vi "subvi_sample_setting.vi"(7 "采样频率":dbl=50000.0 format="%0.2f", 8 "error in":errorcluster caption="错误输入", 11 "physical channel":string="PXI_4499_1/ai0") -> (0 "error out":errorcluster caption="错误输出", 3 "task out":refnum<k21> caption="任务输出")   [LabVIEW 2014]
uses:
  <vilib>/DAQmx/configure/timing.llb/DAQmx Timing (Sample Clock).vi
  <vilib>/DAQmx/create/channels.llb/DAQmx Create Channel (AI-Sound Pressure-Microphone).vi
  <resource>/objmgr/daqmx.rc
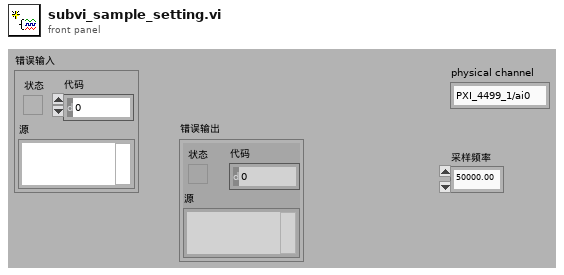
[diagram p1: front panel]
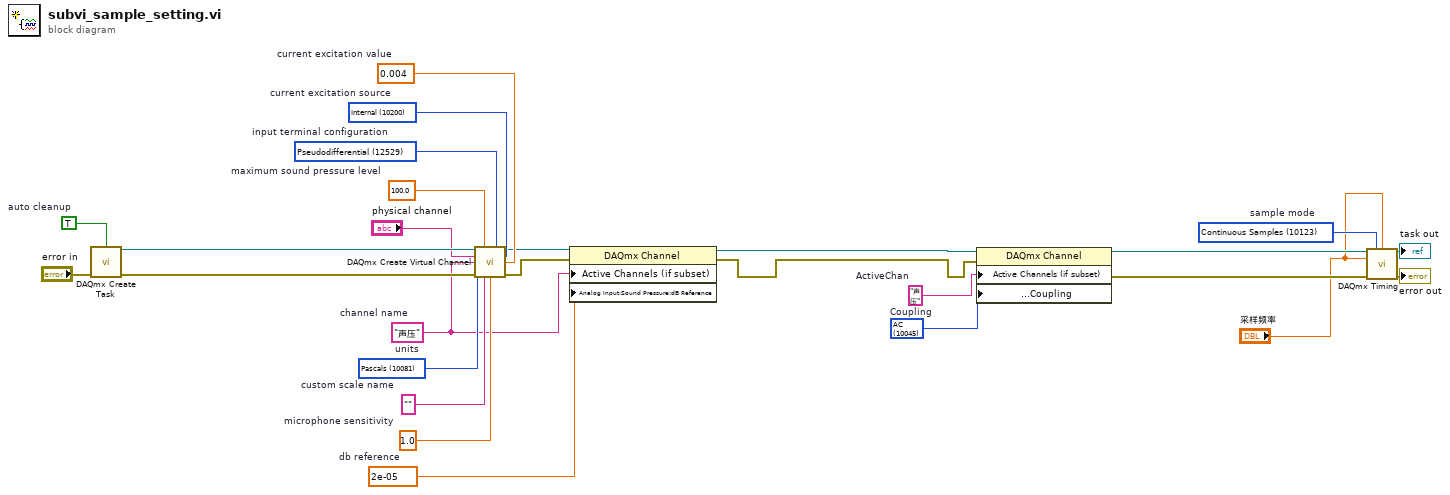
[diagram p0: block diagram]
diagram:
  w2 = 10123 items=["Finite Samples"=10178, "Continuous Samples"=10123, "Hardware Timed Single Point"=12522]  # sample mode
  w8 = 10045 items=["AC"=10045, "DC"=10050, "GND"=10066]  # Coupling
  w9 = "声压"  # ActiveChan
  w11 = 2e-05  # db reference
  w15 = 12529 items=["default"=-1, "RSE"=10083, "NRSE"=10078, "Differential"=10106, "Pseudodifferential"=12529]  # input terminal configuration
  w16 = 10081 items=["Pascals"=10081, "From Custom Scale"=10065]  # units
  w17 = 1.0  # microphone sensitivity
  w18 = 0.004  # current excitation value
  w19 = 10200 items=["Internal"=10200, "External"=10167, "None"=10230]  # current excitation source
  w20 = 100.0  # maximum sound pressure level
  w10 = "声压"  # channel name
  w21 = ""  # custom scale name
  w24 = TRUE  # auto cleanup
  n1 = call <vilib>:"DAQmx Create Task.vi"("auto cleanup"=w24, "error in"="error in") -> ("task out"=w23:refnum<k21>, "error out"=w25:errorcluster)  [unwired: 12 in]
  n2 = call-poly <vilib>:"DAQmx Create Virtual Channel.vi"("task in"=w23, "maximum sound pressure level"=w20, "input terminal configuration"=w15, "physical channels"="physical channel", "current excitation source"=w19, "name to assign"=w10, "current excitation value"=w18, "units"=w16, "error in"=w25, "custom scale name"=w21, "microphone sensitivity"=w17) -> ("task out"=w14:refnum<k21>, "error out"=w13:errorcluster)  [unwired: 3 in]
  n3 = property class="DAQmx Channel"(reference=w14, error in=w13, "Active Channels (if subset)"=w10, "Analog Input:Sound Pressure:dB Reference"=w11) -> (reference out=w6:refnum<k21>, error out=w12:errorcluster)
  n4 = property class="DAQmx Channel"(reference=w6, error in=w12, "Active Channels (if subset)"=w9, "Analog Input:General Properties:Input Configuration:Coupling"=w8) -> (reference out=w3:refnum<k21>, error out=w7:errorcluster)
  n5 = call-poly <vilib>:"DAQmx Timing.vi"("task/channels in"=w3, "sample mode"=w2, "samples per channel"="采样频率", "rate"="采样频率", "error in"=w7) -> ("task out"=→"task out":refnum<k21>, "error out"=→"error out":errorcluster)  [unwired: 9 in]
